vi "AlliGator Enter Power Law Parameters Dialog.vi"(8 "Error In":errorcluster) -> (0 "Error Out":errorcluster, 1 "Cancelled?":bool, 3 "Power Law Parameters out":T1)   [LabVIEW 2021, in "AlliGator Decay Fit Parameter Map.lvlib"]
doc: "Lets the user enter the power law parameters describing the CV_tau(I) dependency, where <B>I</B> is the pixel intensity and <B>CV_tau</B> is the lifetime coefficient of variation obtained from calibration measurements."
uses:
  AlliGator Power Law Parameters.ctl
  AlliGator Decay Fit Parameter Map.lvlib
panel:
  in  "Power Law Parameters":T1
  out "Message":string
  in  "Cancel":bool
  in  "OK":bool
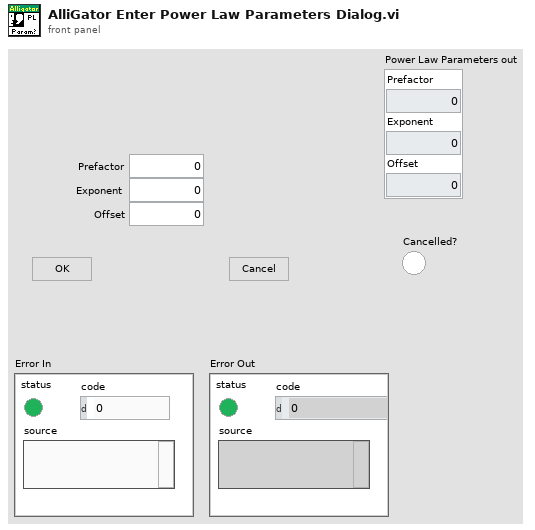
[diagram p1: front panel]
types:
  T1 = typedef "AlliGator Decay Fit Parameter Map.lvlib/AlliGator Power Law Parameters.ctl" = cluster{"Prefactor":dbl, "Exponent":dbl, "Offset":dbl}
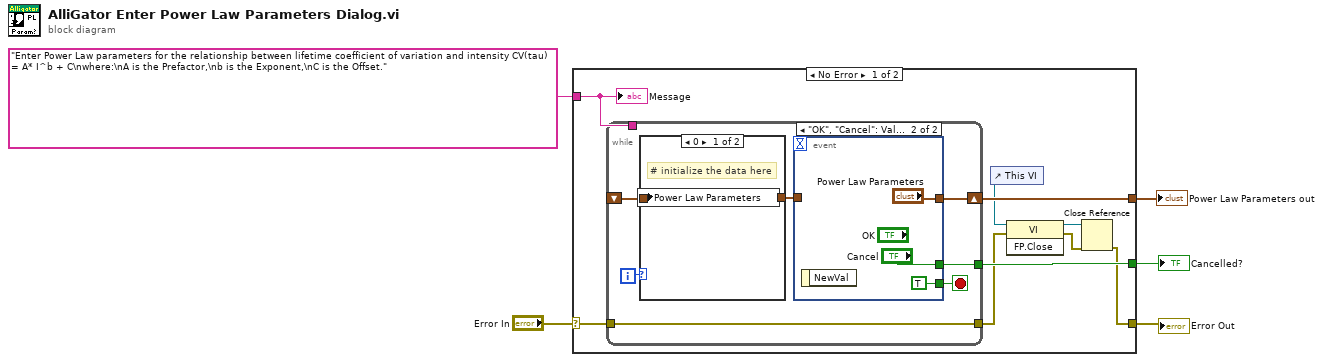
[diagram p0: block diagram]
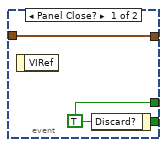
[diagram p3: hidden frame]
diagram:
  n1 = case shown="No Error" "Error In" {
    selector: "Error In" -> [w10 w29]
    tunnel: [w14 _] -> w5
    tunnel: [w13 _] -> w4
    tunnel: "Enter Power Law parameters for the relationship between lifetime coefficient of variation and intensity CV(tau) = A* I^b + C\nwhere:\nA is the Prefactor,\nb is the Exponent,\nC is the Offset." ("Input Message") -> [w12 _]
    tunnel: [w11 w29] -> w2
    frame No Error {
      n2 = while {
        tunnel: [w20] -> w14
        shift-right: [w17] -> w13
        shift-left: _ -> [w18]
        tunnel: w12 -> [_]
        tunnel: w10 -> [w15]
        tunnel: [w15] -> w7
        i -> [w19]
        stop <- w21 stop-if-true
        n3 = case shown="0" w19 {
          tunnel: w18 -> [w22 w23]
          tunnel: [w22 w23] -> w16
          frame 0 {
            # "# initialize the data here"
            n4 = local write "Power Law Parameters"(w22) -> ()
          }
          frame 1, Default {
          }
        }
        n5 = event shown="[1] \"OK\", \"Cancel\": Value Change" {
          selector: _ -> [_ _]
          dyn-events: _ -> [_ _]
          timeout: _ -> [_ _]
          tunnel: [w25 TRUE ("Discard?")] -> w21
          tunnel: [w25 "Cancel"] -> w20
          tunnel: [w24 "Power Law Parameters"] -> w17
          tunnel: w16 -> [w24 _]
          event Panel Close? {
            w25 = TRUE ("Discard?")
            n6 = event-data() -> ()  [unwired: 1 in, 1 out]
            n7 = event-data("Discard?"=w25) -> ()  [unwired: 1 in, 1 out]
          }
          event "OK", "Cancel": Value Change {
            n8 = event-data() -> ()  [unwired: 1 in, 1 out]
          }
        }
      }
      n9 = control-ref of="This VI"() -> (w6:refnum<vi>)
      n10 = invoke class="VI" method="FP.Close"(reference=w6, error in=w7) -> (reference out=w9:refnum<vi>, error out=w8:errorcluster)  [unwired: 1 in, 1 out]
      n11 = Close Reference(reference=w9, error in (no error)=w8) -> (error out=w11:errorcluster)
      "Message" <- w12
    }
    frame Error {
    }
  }
  "Power Law Parameters out" <- w4
  "Cancelled?" <- w5
  "Error Out" <- w2
